vi "teste-valvulas.vi"() -> ()   [LabVIEW 2010]
uses:
  <vilib>/ptbypt/NI_PtbyPt.lvlib
panel:
  in  "Automático":bool
  in  "Duty Cycle %":i32=50 min=0 max=100 step=1
  in  "Frequência":dbl=1.0 min=0.0 max=15.0 step=0.1
  in  "Write to File":bool
  in  "Samples":i32=100
  in  "DAQ Rate":i32=100
  in  "Path":path=path "\\\\baiacu\\aquisicaomatheus/PROTOTIPO/Exp_Matheus/test1.dat"
  in  "Valvula":bool=TRUE
  out "Valvula":bool
  out "Stop\nProgram":bool
  in  "Stop 1":bool
  out "Pressures":cluster{"mean":dbl, "mean":dbl}(graph)={"mean"=13.665465410461849, "mean"=2.334967581184493}
  out "Test Time\n[hh:mm:ss]":timestamp format="%<%H:%M:%S>T"
  in  "Horário de Verão\n(Padrão +1h)":bool=TRUE
  out "Flowrate":cluster{"mean":dbl, "T":dbl}(graph)
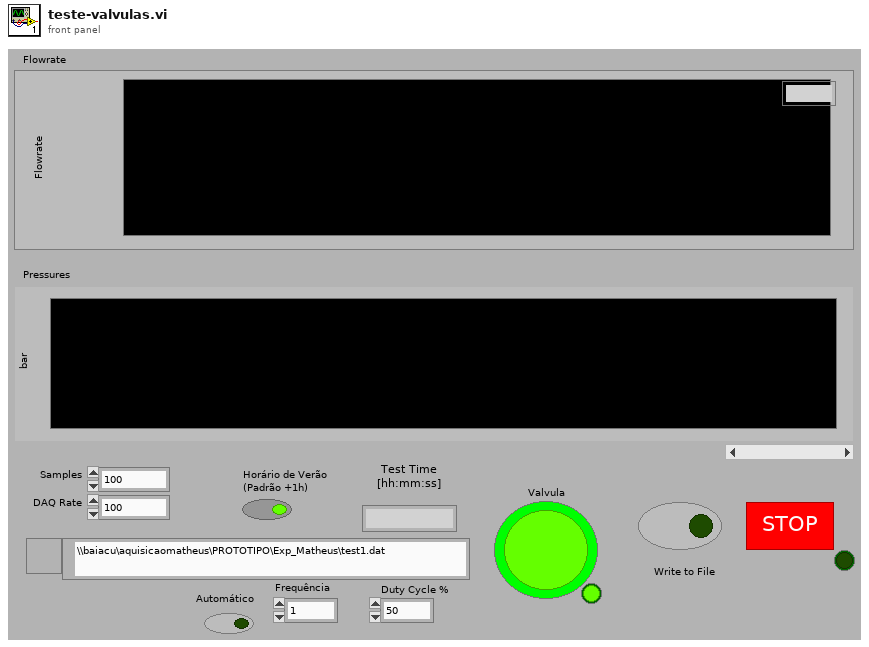
[diagram p1: front panel]
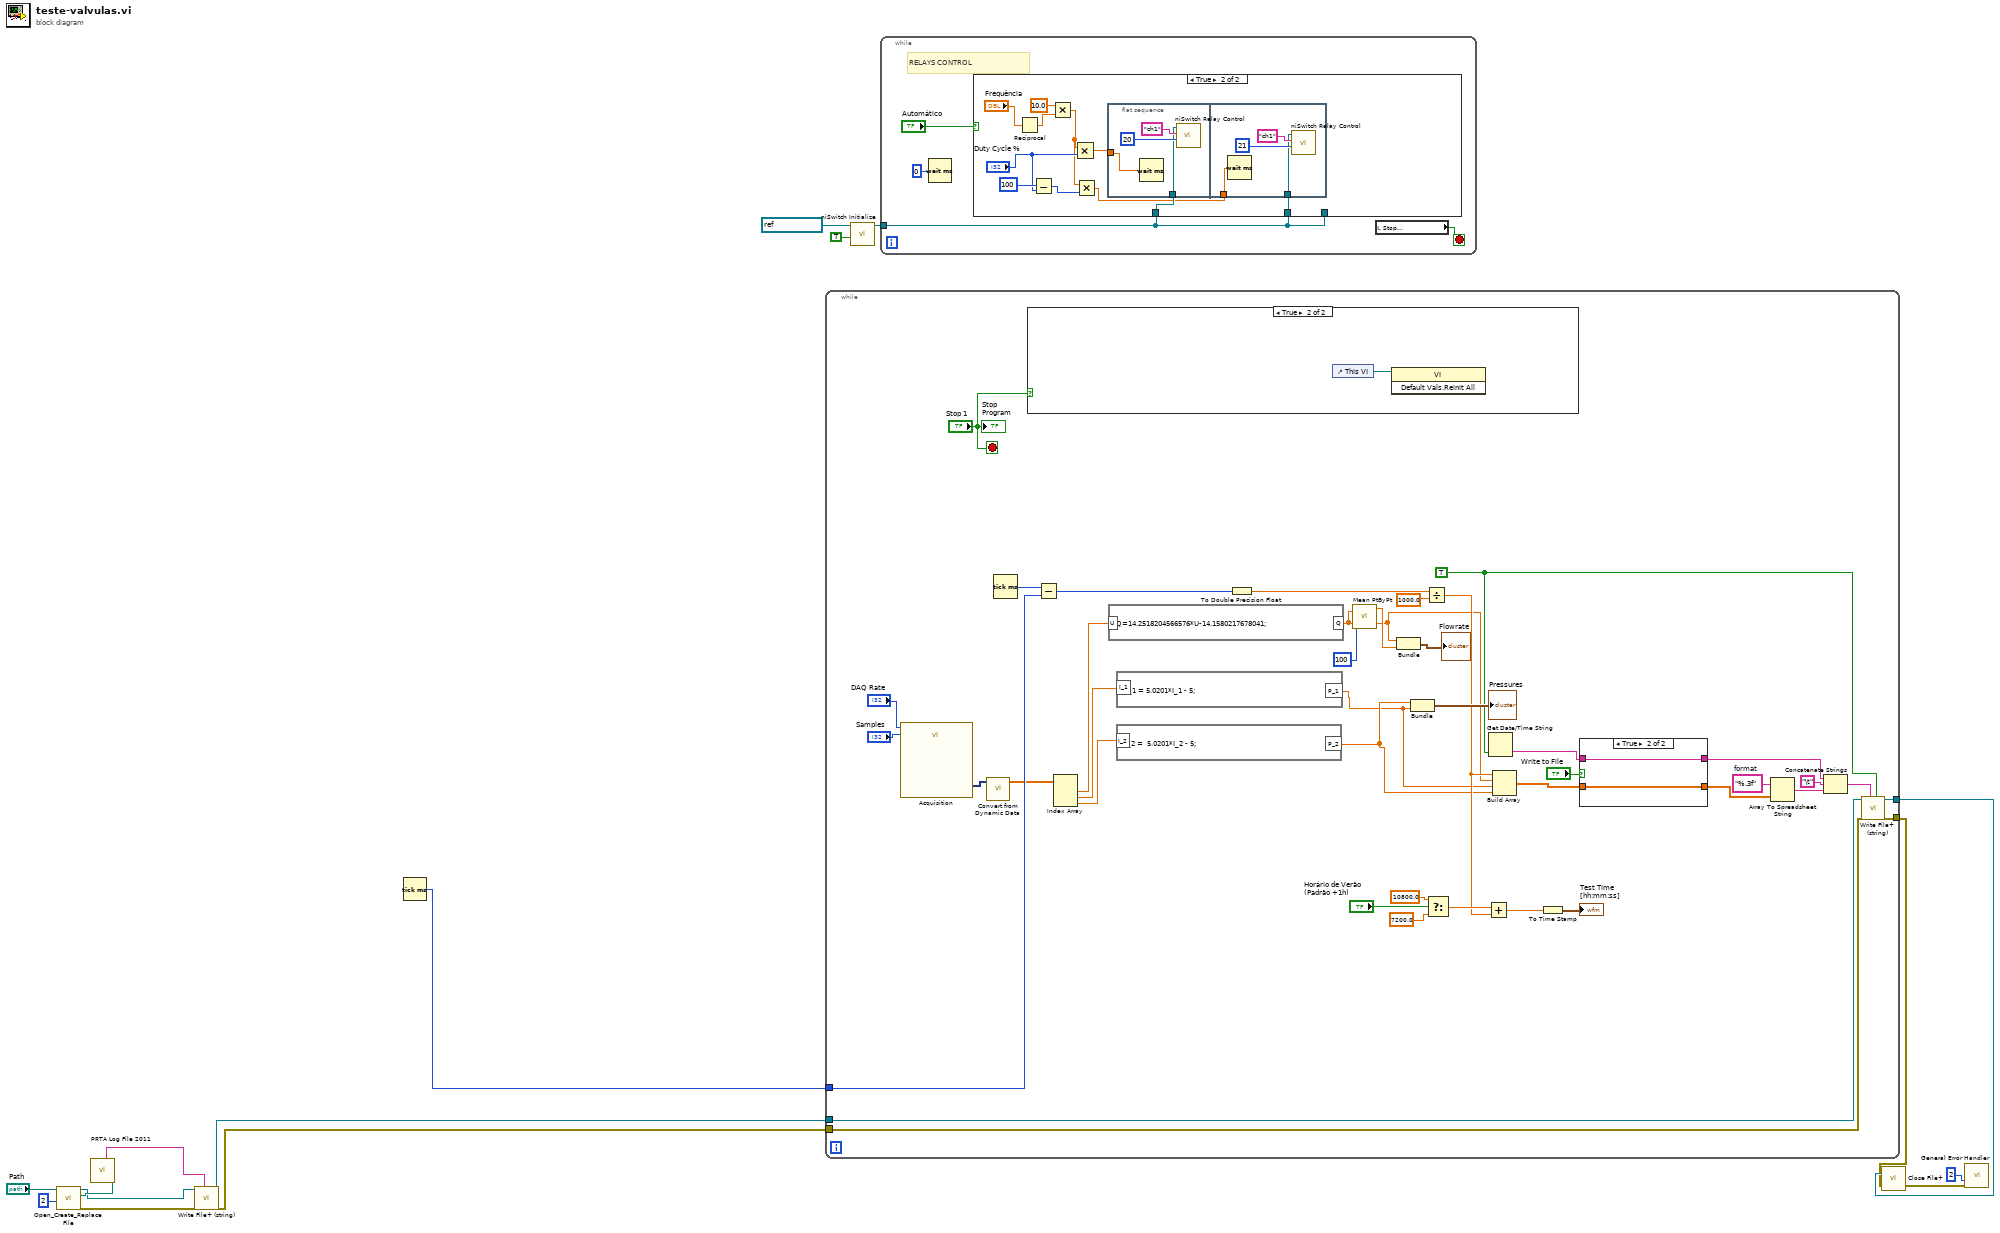
[diagram p0: block diagram]
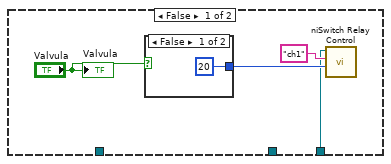
[diagram p2: hidden frame]
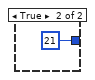
[diagram p3: hidden frame]
diagram:
  n1 = call <vilib>:"Open_Create_Replace File.vi"("function (open:0)"=2, "file path"="Path") -> ("error out"=w9:errorcluster, "new file path"=w12:path, "refnum"=w10:refnum<file>)  [unwired: 4 in, 3 out]
  n2 = call "PRTA Log File 2011.vi"("Output File"=w12) -> ("data file"=w11:string)  [unwired: 7 in]
  n3 = call <vilib>:"Write File+ (string).vi"("string"=w11, "error in (no error)"=w9, "refnum"=w10) -> ("error out"=w5:errorcluster, "dup refnum"=w6:refnum<file>)  [unwired: 3 in, 2 out]
  n4 = Tick Count (ms)() -> (millisecond timer value=w16:u32)
  n5 = while {
    tunnel: w16 -> [w47]
    tunnel: w6 -> [w31]
    tunnel: w5 -> [w30]
    tunnel: [w33] -> w2
    tunnel: [w32] -> w1
    stop <- "Stop 1" stop-if-true
    w39 = "%.3f"  # format
    w36 = TRUE ("want seconds? (F)")
    n6 = call "Acquisition"("rate"="DAQ Rate", "number of samples"="Samples") -> ("data"=w43:dynamicdata)  [unwired: 14 in, 3 out]
    n7 = call "Convert from Dynamic Data"("Dynamic Data Type"=w43) -> ("Array"=w44:dbl[])  [unwired: 3 in]
    n8 = Tick Count (ms)() -> (millisecond timer value=w55:u32)
    n9 = case shown="True" "Stop 1" {
      frame False {
      }
      frame True {
        n10 = control-ref of="This VI"() -> (w60:refnum<vi>)
        n11 = invoke class="VI" method="Default Vals.Reinit All"(reference=w60) -> ()  [unwired: 2 in, 3 out]
      }
    }
    n12 = Subtract(x=w55, y=w47) -> (x-y=w52:u32)
    n13 = Index Array(array=w44) -> (element #1=w57:dbl, element #2=w21:dbl, element #3=w17:dbl)  [unwired: 3 in]
    n14 = formula code="Q=14.2518204566576*U-14.1580217678041;"("U"=w57) -> ("Q"=w23:dbl)
    n15 = formula code="P_2 =  5.0201*I_2 - 5;"("I_2"=w17) -> ("P_2"=w19:dbl)
    n16 = formula code="P_1 = 5.0201*I_1 - 5;"("I_1"=w21) -> ("P_1"=w18:dbl)
    n17 = To Double Precision Float(number=w52) -> (double precision float=w53:dbl)
    n18 = call <vilib>:"Mean PtByPt.vi"("x"=w23, "sample length"=100) -> ("mean"=w24:dbl)  [unwired: 2 in, 1 out]
    n19 = Bundle("Q"=w23, "mean"=w24) -> (→"Flowrate":cluster{"Q":dbl, "mean":dbl})  [unwired: 1 in]
    n20 = Bundle("P_2"=w19, "P_1"=w18) -> (→"Pressures":cluster{"P_2":dbl, "P_1":dbl})  [unwired: 1 in]
    n21 = Divide(x=w53, y=1000.0) -> (x/y=w27:dbl)
    n22 = Select(t=10800.0, s="Horário de Verão\n(Padrão +1h)", f=7200.0) -> (s? t:f=w48:dbl)
    n23 = Add(x=w48, y=w27) -> (x+y=w51:dbl)
    n24 = Get Date/Time String(want seconds? (F)=w36) -> (time string=w35:string)  [unwired: 3 out]
    n25 = Build Array(w27, w23, w18, w19) -> (w34:dbl[])
    n26 = To Time Stamp(1:w51) -> (0:→"Test Time\n[hh:mm:ss]":timestamp)
    n27 = case shown="True" "Write to File" {
      tunnel: w34 -> [_ w59]
      tunnel: [_ w59] -> w41
      tunnel: w35 -> [_ w58]
      tunnel: [_ w58] -> w42
      frame False {
      }
      frame True {
      }
    }
    n28 = Array To Spreadsheet String(array=w41, 3:w39) -> (spreadsheet string=w40:string)  [unwired: 1 out]
    n29 = Concatenate Strings(w42, "\t" ("time string"), w40) -> (w38:string)
    n30 = call <vilib>:"Write File+ (string).vi"("convert eol? (no:F)"=w36, "string"=w38, "error in (no error)"=w30, "refnum"=w31) -> ("error out"=w32:errorcluster, "dup refnum"=w33:refnum<file>)  [unwired: 2 in, 2 out]
    "Stop\nProgram" <- "Stop 1"
  }
  n31 = call <instrlib>:"niSwitch Initialize.vi"("reset device (boolean value)"=TRUE, "resource name"=refnum<k15> "SC1Mod2") -> ("instrument handle out"=w13:refnum<k15>)  [unwired: 8 in, 1 out]
  n32 = while {
    tunnel: w13 -> [w62]
    stop <- w64 stop-if-true
    # "RELAYS CONTROL"
    n33 = Wait (ms)(milliseconds to wait=u32 0) -> ()  [unwired: 1 out]
    n34 = case shown="True" "Automático" {
      tunnel: w62 -> [w65 _]
      tunnel: w62 -> [_ w81]
      tunnel: w62 -> [_ w80]
      frame False {
        n35 = case shown="False" "Valvula" {
          tunnel: [20 21] -> w67
          frame False {
          }
          frame True {
          }
        }
        n36 = call <instrlib>:"niSwitch Relay Control.vi"("relay action (Close Relay)"=w67, "relay name"="ch1" ("String"), "instrument handle"=w65) -> ()  [unwired: 7 in, 2 out]
        "Valvula" <- "Valvula"
      }
      frame True {
        n37 = Reciprocal(x="Frequência") -> (1/x=w78:dbl)
        n38 = Subtract(x=100, y="Duty Cycle %") -> (x-y=w73:i32)
        n39 = Multiply(x=10.0 ("y"), y=w78) -> (x*y=w72:dbl)
        n40 = Multiply(x=w72, y="Duty Cycle %") -> (x*y=w76:dbl)
        n41 = Multiply(x=w72, y=w73) -> (x*y=w71:dbl)
        n42 = flat-sequence {
          tunnel: w81 -> [w83]
          tunnel: w76 -> [w82]
          tunnel: w80 -> [w87]
          tunnel: w71 -> [w86]
          frame #0 {
            n43 = Wait (ms)(milliseconds to wait=w82) -> ()  [unwired: 1 out]
            n44 = call <instrlib>:"niSwitch Relay Control.vi"("relay action (Close Relay)"=20, "relay name"="ch1" ("String"), "instrument handle"=w83) -> ()  [unwired: 7 in, 2 out]
          }
          frame #1 {
            n45 = Wait (ms)(milliseconds to wait=w86) -> ()  [unwired: 1 out]
            n46 = call <instrlib>:"niSwitch Relay Control.vi"("relay action (Close Relay)"=21, "relay name"="ch1" ("String"), "instrument handle"=w87) -> ()  [unwired: 7 in, 2 out]
          }
        }
      }
    }
    n47 = local read "Stop\nProgram"() -> (w64:bool)
  }
  n48 = call <vilib>:"Close File+.vi"("error in (no error)"=w1, "refnum"=w2) -> ("error out"=w3:errorcluster)  [unwired: 1 in, 4 out]
  n49 = call <vilib>:"General Error Handler.vi"("type of dialog (OK msg:1)"=2, "error in (no error)"=w3) -> ()  [unwired: 1 in, 13 out]
